vi "Power ONor OFF(DUT).vi"(7 "String":string, 8 "error in (no error)":errorcluster, 9 "Serial Port Setup":T1={"baud rate"=115200, "data bits"=8, "parity"=enum."None", "stop bits"=10, "flow control"=0} {"flow control" items=["None"=0, "XON/XOFF"=1, "RTS/CTS"=2, "DTR/DSR"=4]; "stop bits" items=["1.0"=10, "1.5"=15, "2.0"=20]; "data bits" min=5 max=8 step=1; "baud rate" items=["75"=75, "110"=110, "134"=134, "150"=150, "300"=300, "600"=600, "1200"=1200, "1800"=1800, "2400"=2400, "4800"=4800, "7200"=7200, "9600"=9600, "14400"=14400, "19200"=19200, "28800"=28800, "38400"=38400, "56000"=56000, "57600"=57600, "115200"=115200, "128000"=128000, "230400"=230400]}, 11 "VISA resource name":refnum<visa-resource-name>="COM3") -> (0 "error out":errorcluster)   [LabVIEW 2019]
uses:
  Control/Serial - Settings.ctl
  <vilib>/Instr/_visa.llb/VISA Configure Serial Port (Instr).vi
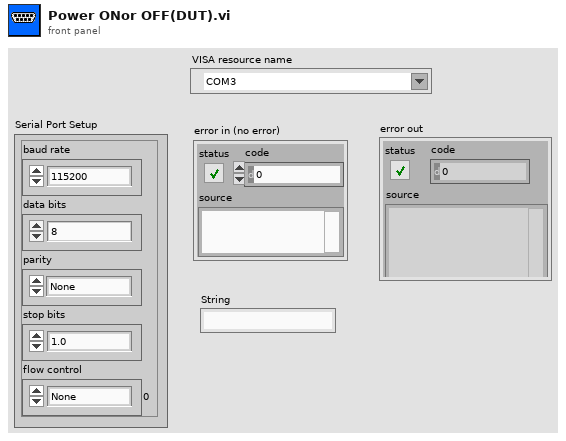
[diagram p1: front panel]
types:
  T1 = typedef "Serial - Settings.ctl" = cluster{"baud rate":u32, "data bits":u16, "parity":enum16{"None", "Odd", "Even", "Mark", "Space"}, "stop bits":u16, "flow control":u16}
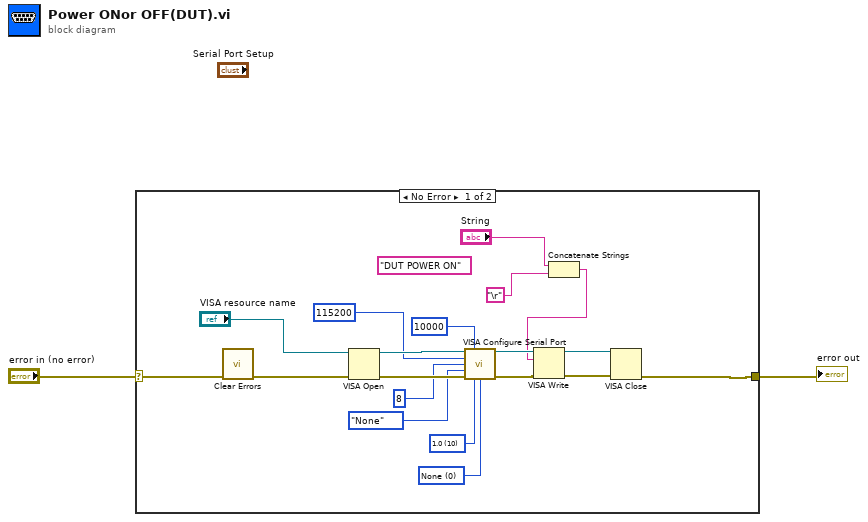
[diagram p0: block diagram]
diagram:
  n1 = case shown="No Error" "error in (no error)" {
    selector: "error in (no error)" -> [w5 w22]
    tunnel: [w3 w22] -> w2
    frame No Error {
      w9 = u16 0 items=["None", "XON/XOFF", "RTS/CTS", "XON/XOFF & RTS/CTS", "DTR/DSR", "XON/XOFF & DTR/DSR"] ("flow control (0:none)")
      w14 = u16 10 items=["1.0"=10, "1.5"=15, "2.0"=20] ("stop bits (10: 1 bit)")
      (unwired) "DUT POWER ON"
      n2 = call <vilib>:"Clear Errors.vi"("error in (no error)"=w5) -> ("error out"=w4:errorcluster)  [unwired: 5 in, 1 out]
      n3 = VISA Open(error in (no error)=w4, VISA resource name="VISA resource name") -> (VISA resource name=w21:refnum<visa-resource-name>, error out=w20:errorcluster)  [unwired: 3 in]
      n4 = call-poly "VISA Configure Serial Port"("VISA resource name"=w21, "timeout (10sec)"=u32 10000, "baud rate (9600)"=u32 115200, "data bits (8)"=u16 8, "parity (0:none)"=enum16{"None", "Odd", "Even", "Mark", "Space"}."None", "error in (no error)"=w20, "stop bits (10: 1 bit)"=w14, "flow control (0:none)"=w9) -> ("VISA resource name out"=w17:refnum<visa-resource-name>, "error out"=w16:errorcluster)  [unwired: 6 in]
      n5 = Concatenate Strings("String", "\r") -> (w7:string)
      n6 = VISA Write(VISA resource name=w17, write buffer=w7, error in (no error)=w16) -> (VISA resource name out=w13:refnum<visa-resource-name>, error out=w12:errorcluster)  [unwired: 1 out]
      n7 = VISA Close(VISA resource name=w13, error in (no error)=w12) -> (error out=w3:errorcluster)
    }
    frame Error {
    }
  }
  "error out" <- w2
